vi "Initialise.vi"(8 "error in (no error)":errorcluster, 10 "System In":refnum<class "abs_System.lvclass">, 11 "Node in":refnum<class "abs_Parallel.lvclass">) -> (0 "error out":errorcluster, 2 "System Out":refnum<class "abs_System.lvclass">, 3 "Node out":refnum<class "abs_Parallel.lvclass">)   [LabVIEW 2021, in "BT.lvlib" / "abs_Parallel.lvclass"]
uses:
  abs_Parallel.lvclass
  C:/Users/Tim/Documents/GitHub/LV_Behaviour_Tree/Source/abs_Composite/abs_Composite.lvclass
  abs_System/abs_System.lvclass
  abs_Node/Status.ctl
  abs_Composite/abs_Composite.lvclass/abs_Composite.ctl
  abs_Parallel.lvclass/abs_Parallel.ctl
  abs_Composite/Properties/Read Num Nodes.vi
  abs_Composite/abs_Composite.lvclass
  abs_Node/abs_Node.lvclass
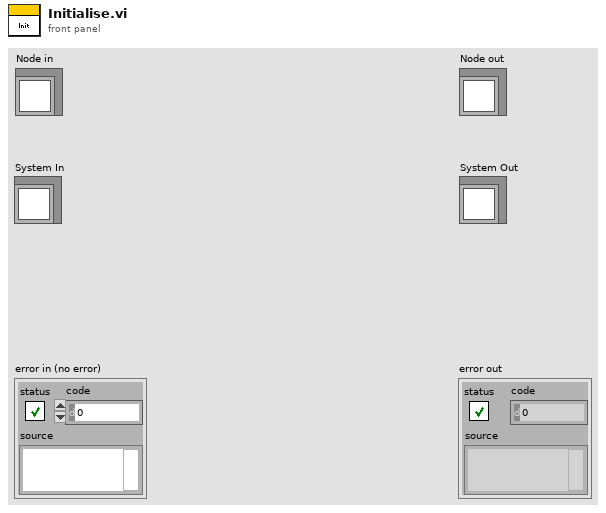
[diagram p1: front panel]
types:
  T1 = typedef "BT.lvlib/abs_Node.lvclass/Status.ctl" = enum16{"Success", "Failure", "Running"}
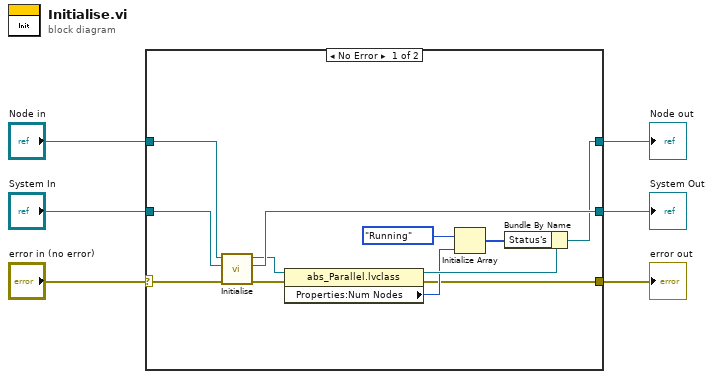
[diagram p0: block diagram]
diagram:
  n1 = case shown="No Error" "error in (no error)" {
    selector: "error in (no error)" -> [w17 w21]
    tunnel: [w9 w21] -> w3
    tunnel: [w18 w20] -> w2
    tunnel: [w11 w19] -> w1
    tunnel: "System In" -> [w16 w20]
    tunnel: "Node in" -> [w15 w19]
    frame No Error {
      n2 = call-parent "Initialise.vi"("error in (no error)"=w17, "System In"=w16, "Node in"=w15) -> ("error out"=w14:errorcluster, "System Out"=w18:refnum<class "abs_System.lvclass">, "Node out"=w13:refnum<class "abs_Parallel.lvclass">)  [unwired: 6 in]
      n3 = property class="abs_Parallel.lvclass"(reference=w13, error in=w14) -> (reference out=w12:refnum<class "abs_Parallel.lvclass">, error out=w9:errorcluster, "Properties:Num Nodes"=w10:i32)
      n4 = Initialize Array(Status."Running" ("Status"), w10) -> (w7:T1[])
      n5 = Bundle By Name(cluster=w12, "Status's"=w7) -> (w11:refnum<class "abs_Parallel.lvclass">)
    }
    frame Error {
    }
  }
  "error out" <- w3
  "Node out" <- w1
  "System Out" <- w2
